vi "Feedback_while.vi"() -> ()   [LabVIEW 2024]
panel:
  out "Numeric 2":i32
  in  "Numeric":dbl
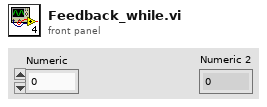
[diagram p1: front panel]
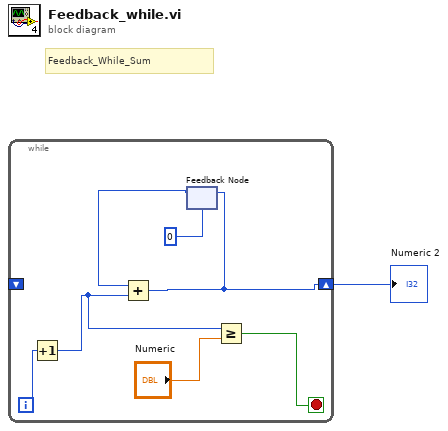
[diagram p0: block diagram]
diagram:
  # "Feedback_While_Sum"
  n1 = while {
    shift-right: [w4] -> w1
    shift-left: _ -> [_]
    i -> [w6]
    stop <- w7 stop-if-true
    n2 = Increment(x=w6) -> (x+1=w5:i32)
    n3 = feedback #1(0) -> (w3:i32)
    n4 = Add(x=w3, y=w5) -> (x+y=w4:i32)
    n5 = feedback-in #1(w4) -> ()
    n6 = Greater Or Equal?(x=w5, y="Numeric") -> (x >= y?=w7:bool)
  }
  "Numeric 2" <- w1
